vi "reorderFIFOdata.vi"(9 "pointsPerLine":i32, 10 "numLines":i32, 11 "inputElements":sgl[](array[numeric])) -> (3 "Reshaped":sgl[][][][](array[numeric]))   [LabVIEW 2016]
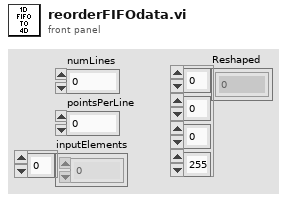
[diagram p1: front panel]
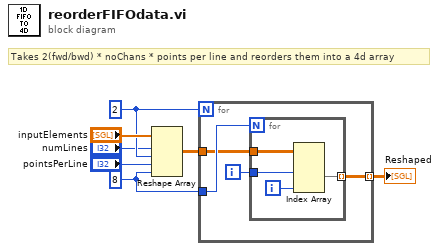
[diagram p0: block diagram]
diagram:
  w4 = 8 ("dimension size")
  w5 = 2 ("dimension size")
  # "Takes 2(fwd/bwd) * noChans * points per line and reorders them into a 4d array"
  n1 = Reshape Array("inputElements", "numLines", w5, "pointsPerLine", w4) -> (w3:sgl[][][][])
  n2 = for {
    N: w5 -> [_]
    tunnel: w3 -> [w9]
    tunnel: w4 -> [w10]
    tunnel: [w8] -> w6 mode=indexing
    i -> [w11]
    n3 = for {
      N: w10 -> [_]
      tunnel: w9 -> [w13]
      tunnel: w11 -> [w15]
      tunnel: [w12] -> w8 mode=indexing
      i -> [w14]
      n4 = Index Array(array=w13, index (dim 1)=w15, index (dim 3)=w14) -> (element=w12:sgl[][])  [unwired: 2 in]
    }
  }
  "Reshaped" <- w6
